vi "DisplayTemperaturesFVIR.vi"(0 "Raw SRI Data":string[](array[string]), 3 "error in":errorcluster) -> (7 "SRI Butane Levels":string[][](array[string]), 10 "error out":errorcluster)   [LabVIEW 2020, in "Modbus.lvlib"]
uses:
  Modbus/Modbus.lvlib
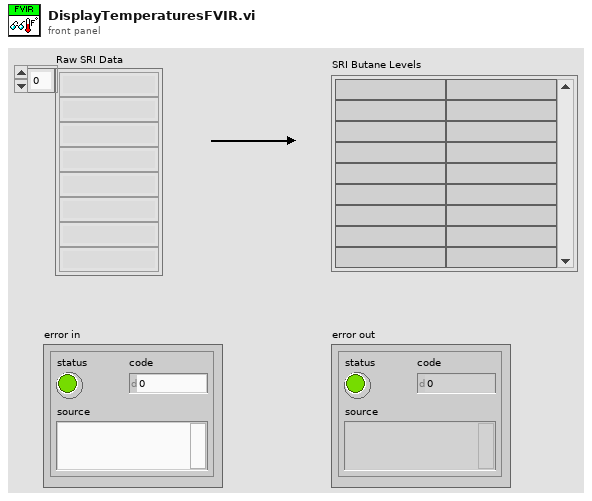
[diagram p1: front panel]
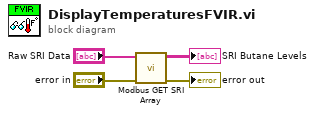
[diagram p0: block diagram]
diagram:
  n1 = call "Modbus GET SRI Array.vi"("error in"="error in", "Raw SRI Data in"="Raw SRI Data") -> ("error out"=→"error out":errorcluster, "SRI Butane Levels"=→"SRI Butane Levels":string[][])  [unwired: 8 in]
